vi "Set main screen FOV control index.vi"(8 "error in (no error)":errorcluster, 11 "FOV control index":i32) -> (0 "error out":errorcluster)   [LabVIEW 2017]
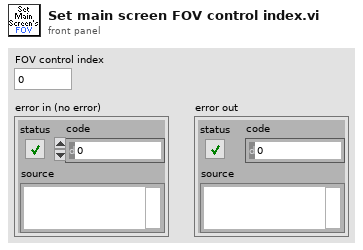
[diagram p1: front panel]
types:
  T1 = typedef "FOV values cluster.ctl" = cluster{"Norm value":sgl, "FOV text":string, "FOV value":i32, "All FOV values":i32[], "All norm FOV values":sgl[], "All FOV value strings":string[], "Strings And Values []":T2}
  T2 = typedef "LVStringsAndValuesArrayTypeDef_SGL.ctl" = cluster{"String":string, "Value":sgl}[]
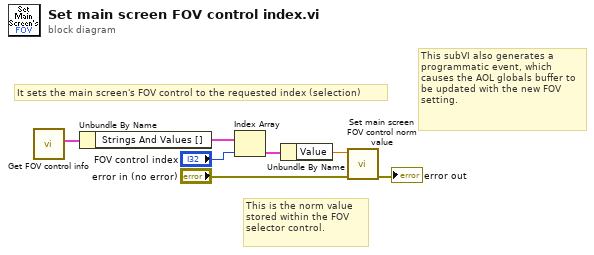
[diagram p0: block diagram]
diagram:
  # "This subVI also generates a programmatic event, which causes the AOL globals buffer to be updated with the new FOV setting."
  # "This is the norm value\nstored within the FOV selector control."
  # "It sets the main screen's FOV control to the requested index (selection)"
  n1 = call "Get FOV control info.vi"() -> ("FOV values cluster"=w1:T1)  [unwired: 8 in, 3 out]
  n2 = Unbundle By Name(w1) -> ("Strings And Values []"=w6:T2)
  n3 = Index Array(array=w6, index="FOV control index") -> (element=w5:cluster{"String":string, "Value":sgl})
  n4 = Unbundle By Name(w5) -> ("Value"=w7:sgl)
  n5 = call "Set main screen FOV control norm value.vi"("error in (no error)"="error in (no error)", "FOV norm value! (Signaling)"=w7) -> ("error out"=→"error out":errorcluster)  [unwired: 9 in]
